vi "Planta_LazoAbierto.vi"() -> ()   [LabVIEW 2012]
panel:
  out "Entrada":dbl=1.9246659085973719
  in  "b1":dbl=1.0
  in  "b2":dbl=-1.628
  in  "b3":dbl=0.6649
  in  "a1":dbl
  in  "a2":dbl=69.06
  in  "a3":dbl=0.001401
  in  "tiempo":i32=100
  in  "u(k-2)":dbl
  in  "u(k-1)":dbl
  in  "Entrada Deseada":dbl(knob)=1.9246659085973719 scale=0.0..3.0
  in  "Y(k-2)":dbl
  in  "Y(k-1)":dbl
  out "Waveform Chart":dbl(graph)=3602.171386268788
  # "MODELO DE LA PLANTA"
  # "Z  +"
  # "Z^2  +"
  # "Gp(z) = --------------------------------------------------------"
  # "Z^2  +"
  # "Z  +"
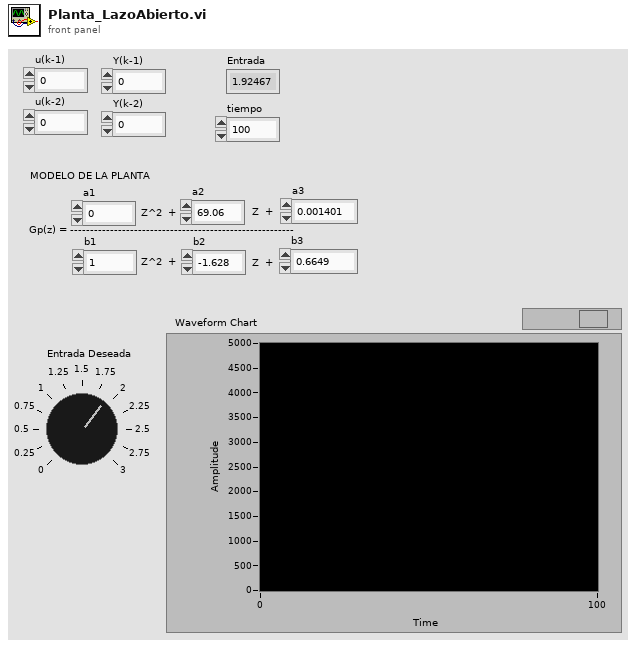
[diagram p1: front panel]
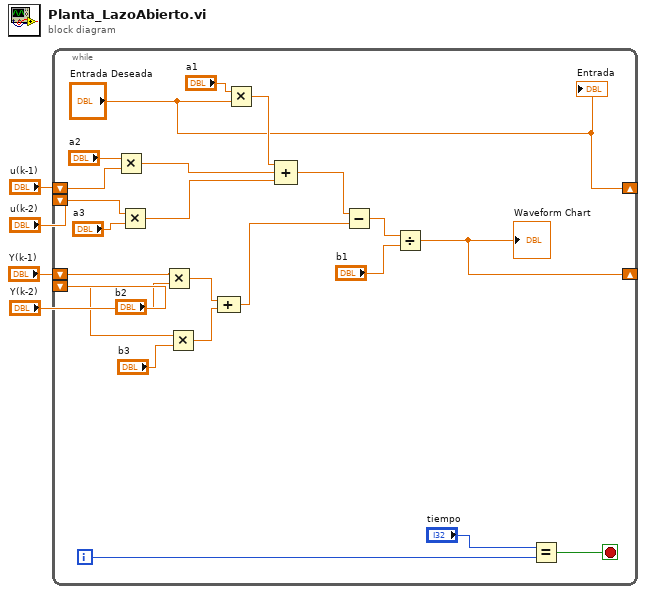
[diagram p0: block diagram]
diagram:
  n1 = while {
    shift-right: [w7] -> _
    shift-left: "Y(k-1)" -> [w16]
    shift-left: "Y(k-2)" -> [w15]
    shift-right: ["Entrada Deseada"] -> _
    shift-left: "u(k-1)" -> [w23]
    shift-left: "u(k-2)" -> [w21]
    i -> [w26]
    stop <- w25 stop-if-true
    n2 = Multiply(x="a2", y=w23) -> (x*y=w19:dbl)
    n3 = Multiply(x=w21, y="a3") -> (x*y=w18:dbl)
    n4 = Multiply(x=w16, y="b2") -> (x*y=w13:dbl)
    n5 = Multiply(x=w15, y="b3") -> (x*y=w12:dbl)
    n6 = Compound Arithmetic op=ADD(w13, w12) -> (w10:dbl)
    n7 = Multiply(x="a1", y="Entrada Deseada") -> (x*y=w6:dbl)
    n8 = Compound Arithmetic op=ADD(w6, w19, w18) -> (w11:dbl)
    n9 = Subtract(x=w11, y=w10) -> (x-y=w9:dbl)
    n10 = Divide(x=w9, y="b1") -> (x/y=w7:dbl)
    "Waveform Chart" <- w7
    n11 = Equal?(x="tiempo", y=w26) -> (x = y?=w25:bool)
    "Entrada" <- "Entrada Deseada"
  }
